vi "Extract Enum Segments.vi"(7 "Start Index":i32, 8 "error in (no error)":errorcluster, 10 "Segments in":T1[](array[typedef]), 11 "ProtoParser in":refnum<class "ProtoParser.lvclass">) -> (0 "error out":errorcluster, 1 "Enumeration Segments":T1[](array[typedef]), 2 "Remaining":T1[](array[typedef]), 3 "ProtoParser out":refnum<class "ProtoParser.lvclass">, 5 "Next Index":i32)   [LabVIEW 2020, in "LV-Protoc.lvlib" / "ProtoParser.lvclass"]
uses:
  ProtoParser.lvclass
  Segment Type.ctl
  LV-Protoc.lvlib
  Raw Segment.ctl
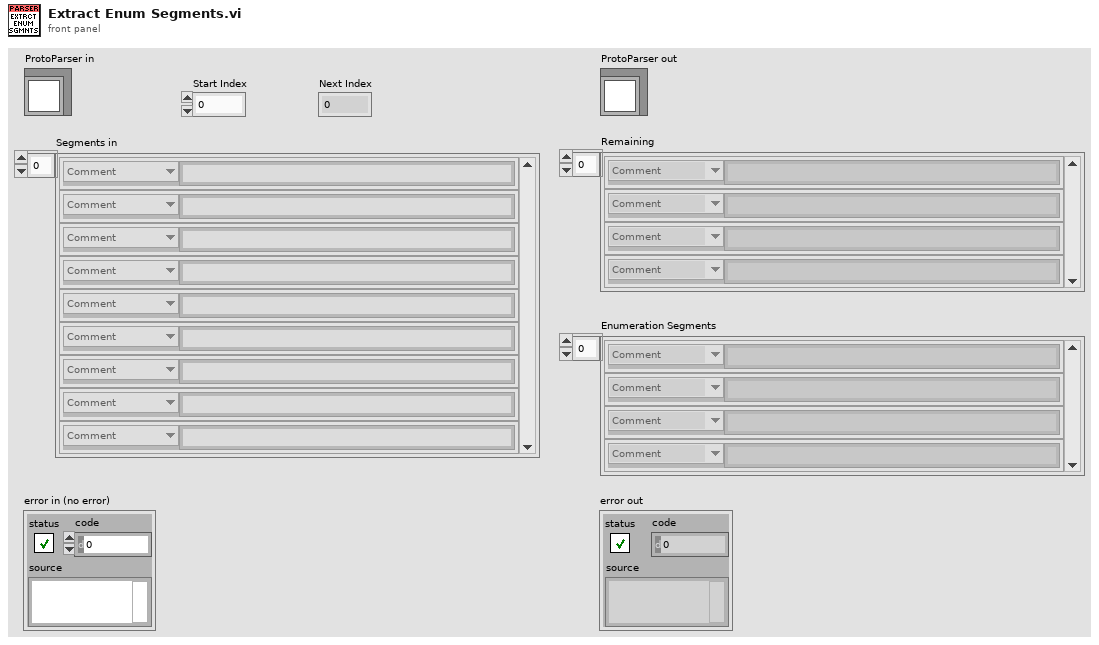
[diagram p1: front panel]
types:
  T1 = typedef "LV-Protoc.lvlib/Raw Segment.ctl" = cluster{"Type":T2, "Text":string}
  T2 = typedef "LV-Protoc.lvlib/Segment Type.ctl" = enum16{"Comment", "Message Open", "Enum Open", "Message Close", "Enum Close", "Field", "Syntax", "Import", "Enum Value", "Package", "Reserved"}
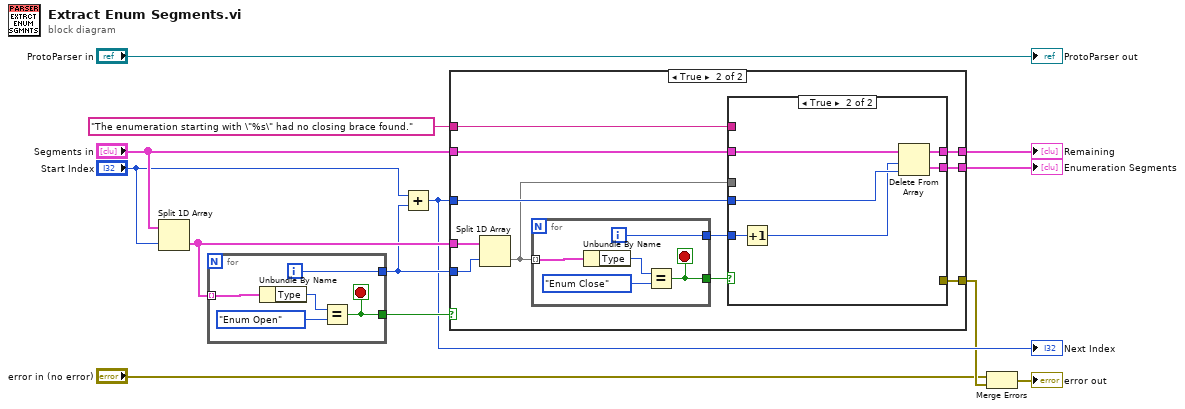
[diagram p0: block diagram]
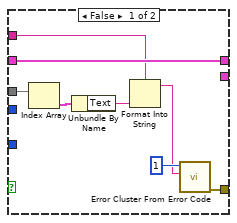
[diagram p3: hidden frame]
diagram:
  n1 = Split 1D Array(array="Segments in", index="Start Index") -> (second subarray=w13:T1[])  [unwired: 1 out]
  n2 = for {
    tunnel: w13 -> [w18] mode=indexing
    tunnel: [w15] -> w8
    tunnel: [w14] -> w12
    i -> [w15]
    stop <- w14 stop-if-true
    n3 = Unbundle By Name(w18) -> ("Type"=w17:T2)
    n4 = Equal?(x=w17, y=Segment_Type."Enum Open") -> (x = y?=w14:bool)
  }
  n5 = Add(x="Start Index", y=w8) -> (x+y=w5:i32)
  "Next Index" <- w5
  n6 = case shown="True" w12 {
    tunnel: w13 -> [_ w30]
    tunnel: w8 -> [_ w25]
    tunnel: "Segments in" -> [w19 w26]
    tunnel: [w19 w27] -> w9
    tunnel: w5 -> [_ w24]
    tunnel: [_ w23] -> w6
    tunnel: "The enumeration starting with \"%s\" had no closing brace found." -> [_ w21]
    tunnel: [_ w20] -> w3
    frame False {
    }
    frame True {
      n7 = Split 1D Array(array=w30, index=w25) -> (second subarray=w22:T1[])  [unwired: 1 out]
      n8 = for {
        tunnel: w22 -> [w49] mode=indexing
        tunnel: [w46] -> w28
        tunnel: [w45] -> w29
        i -> [w46]
        stop <- w45 stop-if-true
        n9 = Unbundle By Name(w49) -> ("Type"=w48:T2)
        n10 = Equal?(x=w48, y=Segment_Type."Enum Close") -> (x = y?=w45:bool)
      }
      n11 = case shown="True" w29 {
        tunnel: w28 -> [_ w40]
        tunnel: [w38 w42] -> w27
        tunnel: w26 -> [w38 w44]
        tunnel: w24 -> [_ w43]
        tunnel: [_ w41] -> w23
        tunnel: w22 -> [w36 _]
        tunnel: w21 -> [w33 _]
        tunnel: [w31 _] -> w20
        frame False {
          n12 = Index Array(array=w36) -> (element=w35:T1)  [unwired: 1 in]
          n13 = Unbundle By Name(w35) -> ("Text"=w34:string)
          n14 = Format Into String(format string=w33, w34) -> (resulting string=w32:string)  [unwired: 2 in, 1 out]
          n15 = call <vilib>:"Error Cluster From Error Code.vi"("error message (\"\")"=w32, "error code (0)"=1) -> ("error out"=w31:errorcluster)  [unwired: 7 in]
        }
        frame True {
          n16 = Increment(x=w40) -> (x+1=w39:i32)
          n17 = Delete From Array(array=w44, length=w39, index=w43) -> (deleted portion=w41:T1[], array with subset deleted=w42:T1[])
        }
      }
    }
  }
  "Enumeration Segments" <- w6
  "Remaining" <- w9
  n18 = Merge Errors("error in (no error)", w3) -> (→"error out":errorcluster)
  "ProtoParser out" <- "ProtoParser in"
